vi "Register Abortable.vi"(8 "error in (no error)":errorcluster, 9 "Task ID":string, 10 "EnQr":refnum<class "Message Enqueuer.lvclass">, 11 "AbortManager in":refnum<class "AbortManager.lvclass">) -> (0 "error out":errorcluster, 3 "AbortManager out":refnum<class "AbortManager.lvclass">)   [LabVIEW 2020, in "Volatus.lvlib" / "AbortManager.lvclass"]
uses:
  AbortManager.lvclass
  <vilib>/ActorFramework/Message Enqueuer/Message Enqueuer.lvclass
  AbortManager.lvclass/AbortManager.ctl
  AbortHandler Messages/Abort Msg/Abort Msg.lvclass
  <vilib>/ActorFramework/Message Enqueuer/Message Priority.ctl
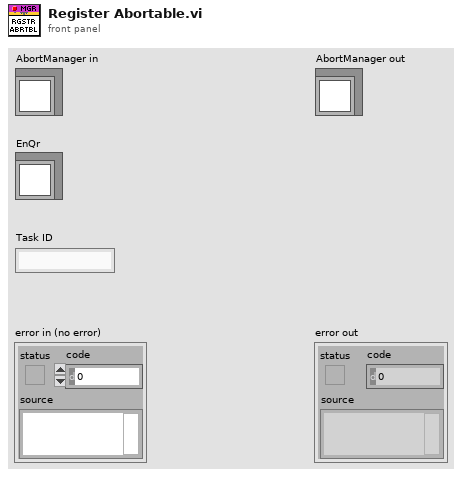
[diagram p1: front panel]
types:
  T1 = map{string, refnum<class "Message Enqueuer.lvclass">}
  T2 = typedef "Actor Framework.lvlib/Message Enqueuer.lvclass/Message Priority.ctl" = enum16{"Low", "Normal", "High"}
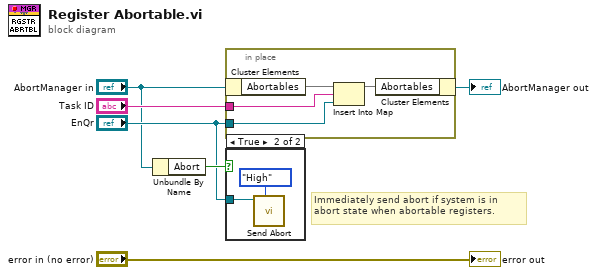
[diagram p0: block diagram]
diagram:
  # "Immediately send abort if system is in abort state when abortable registers."
  n1 = Unbundle By Name("AbortManager in") -> ("Abort"=w3:bool)
  n2 = in-place {
    in-place-border: "Task ID" -> [w9]
    in-place-border: "EnQr" -> [w8]
    n3 = in-place-cluster #1("AbortManager in") -> ("Abortables"=w10:T1)
    n4 = Insert Into Map(map in=w10, key=w9, value=w8) -> (map out=w7:T1)  [unwired: 2 out]
    n5 = in-place-cluster #1("Abortables"=w7) -> (→"AbortManager out":refnum<class "AbortManager.lvclass">)
  }
  n6 = case shown="True" w3 {
    tunnel: "EnQr" -> [_ w12]
    frame False {
    }
    frame True {
      n7 = call "Send Abort.vi"("Message Priority (Normal)"=Message_Priority."High", "Message Enqueuer"=w12) -> ()  [unwired: 8 in, 2 out]
    }
  }
  "error out" <- "error in (no error)"
